vi "Calculate Digital to Analog Converter Latency.vi"() -> ()   [LabVIEW 2013]
uses:
  <vilib>/rvi/interface/common/niFpgaWaitOnOcc.vi
  <vilib>/FPGAPlugInAG/PCIe-1473R/niLvFpga_Open_PCIe-1473R.vi
  <vilib>/rvi/interface/common/dynamic/niFpgaDynamicAddResources.vi
  <vilib>/FPGAPlugInAG/Dynamic/niLvFpga_Reset_Dynamic.vi
  <vilib>/FPGAPlugInAG/Dynamic/niLvFpga_Run_Dynamic.vi
  <vilib>/Utility/error.llb/Error Cluster From Error Code.vi
  <vilib>/rvi/errors/niLvFpgaAdjustHostInterfaceError.vi
  <vilib>/rvi/interface/nirviOpenFPGA/nirviOpenFPGA.xnode
  FPGA Bitfiles/Digital_To_Analog_Latency_Test.lvbitx
  <vilib>/rvi/interface/nirviMethod/nirviMethod.xnode
  <vilib>/rvi/interface/nirviReadWriteControl/nirviReadWriteControl.xnode
  NiFpgaLv.dll
  <vilib>/rvi/interface/Simulation/niFpgaSimulationCallBeginRW.vi
panel:
  out "error out":errorcluster
  out "Latency(Secs)":dbl
  in  "On":bool
  in  "frequency (Hz)":dbl=1000.0
  in  "stop":bool
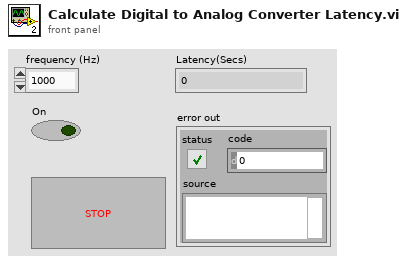
[diagram p1: front panel]
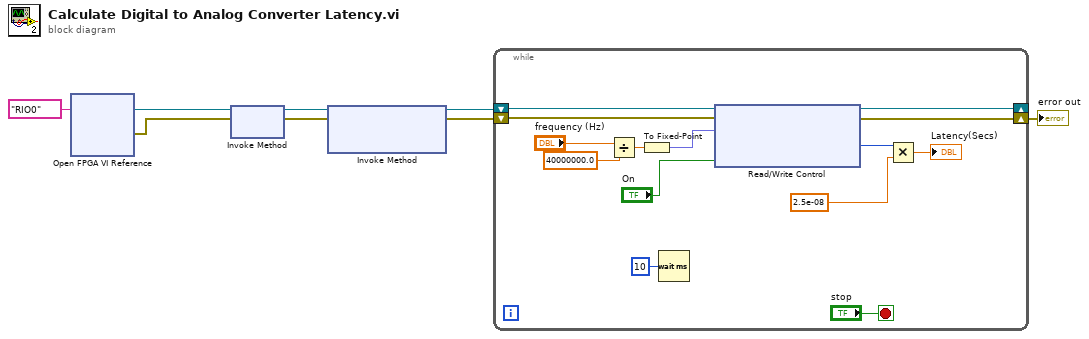
[diagram p0: block diagram]
diagram:
  n1 = xnode "Open FPGA VI Reference"("resource name"=tag "RIO0") -> ("FPGA VI Reference Out"=w7:refnum<k20>, "error out"=w4:errorcluster)  [unwired: 1 in]
  n2 = xnode "Invoke Method"("FPGA VI Reference In"=w7, "error in"=w4) -> ("FPGA VI Reference Out"=w6:refnum<k20>, "error out"=w3:errorcluster)
  n3 = xnode "Invoke Method"("FPGA VI Reference In"=w6, "error in"=w3) -> ("FPGA VI Reference Out"=w5:refnum<k20>, "error out"=w2:errorcluster)  [unwired: 1 in]
  n4 = while {
    shift-right: [w11] -> _
    shift-left: w5 -> [w20]
    shift-right: [w10] -> w1
    shift-left: w2 -> [w9]
    stop <- "stop" stop-if-true
    n5 = Divide(x="frequency (Hz)", y=40000000.0) -> (x/y=w17:dbl)
    n6 = To Fixed-Point(number=w17) -> (fixed-point=w16:fxp<+,32,0>)  [unwired: 1 in]
    n7 = Wait (ms)(milliseconds to wait=u32 10) -> ()  [unwired: 1 out]
    n8 = xnode "Read/Write Control"("FPGA VI Reference In"=w20, "error in"=w9, "frequency (periods/tick)"=w16, "On"="On") -> ("FPGA VI Reference Out"=w11:refnum<k20>, "error out"=w10:errorcluster, "Ticks Elapsed"=w14:u32)
    n9 = Multiply(x=w14, y=2.5e-08) -> (x*y=→"Latency(Secs)":dbl)
  }
  "error out" <- w1
